vi "Draw Regular Polygon.vi"(6 "Draw Para":T2={"fill?(F)"=TRUE, "color(black)"=0, "pen"={"Width"=1, "Style"=enum."Solid"}}, 8 "错误输入":errorcluster, 9 "Para":T1={"Radius"=10, "Divisions"=4, "Closed"=TRUE}, 10 "Center":T3, 11 "Pic in":picture) -> (0 "错误输出":errorcluster, 3 "Pic out":picture)   [LabVIEW 2012, in "Picture Box Tools.lvlib" / "Basic Shape.lvlib"]
uses:
  Basic Shape.lvlib
  Point Custom Control.ctl
  Draw Para Custom Control.ctl
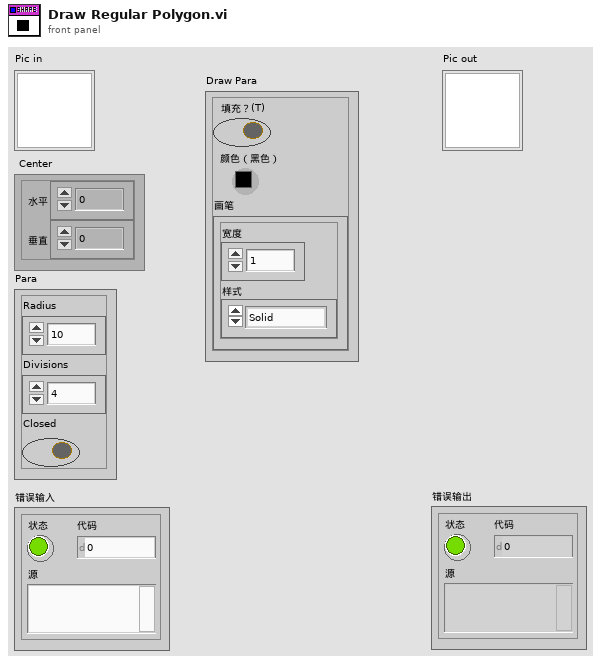
[diagram p1: front panel]
types:
  T1 = cluster{"Radius":i16, "Divisions":i16, "Closed":bool}
  T2 = typedef "Picture Box Tools.lvlib/Basic Shape.lvlib/Draw Para Custom Control.ctl" = cluster{"fill?(F)":bool, "color(black)":u32, "pen":cluster{"Width":u16, "Style":enum32{"Solid", "Dash", "Dot", "DashDot", "DashDotDot"}}}
  T3 = typedef "Picture Box Tools.lvlib/Basic Shape.lvlib/Point Custom Control.ctl" = cluster{"horizontal":i16, "vertical":i16}
  T4 = cluster{"Width":u16, "Style":enum32{"Solid", "Dash", "Dot", "DashDot", "DashDotDot"}}
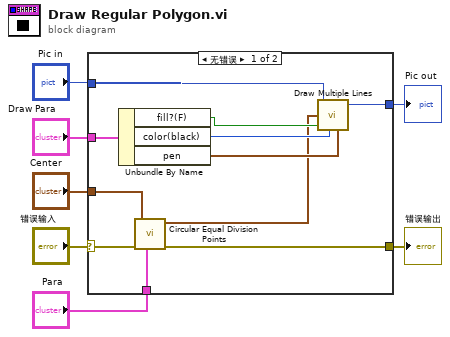
[diagram p0: block diagram]
diagram:
  n1 = case shown="无错误" "错误输入" {
    selector: "错误输入" -> [w18 w20]
    tunnel: [w17 w20] -> w6
    tunnel: "Para" -> [w11 _]
    tunnel: "Center" -> [w15 _]
    tunnel: "Pic in" -> [w10 w19]
    tunnel: [w16 w19] -> w2
    tunnel: "Draw Para" -> [w14 _]
    frame No Error {
      n2 = Unbundle By Name(w14) -> ("fill?(F)"=w9:bool, "color(black)"=w12:u32, "pen"=w13:T4)
      n3 = call "Circular Equal Division Points.vi"("Para"=w11, "错误输入"=w18, "Center"=w15) -> ("错误输出"=w17:errorcluster, "Absolute Point Array"=w8:T3[])  [unwired: 6 in, 1 out]
      n4 = call <vilib>:"Draw Multiple Lines.vi"("picture"=w10, "line endpoints"=w8, "fill?(F)"=w9, "color(black)"=w12, "pen"=w13) -> ("new picture"=w16:picture)  [unwired: 4 in]
    }
    frame Error {
    }
  }
  "Pic out" <- w2
  "错误输出" <- w6
